vi "Set Framed Sensor Path.vi"(8 "error in (no error)":errorcluster, 10 "Framed Sensor Path":path, 11 "Sensor Model in":refnum<class "Sensor Model.lvclass">) -> (0 "error out":errorcluster, 3 "Sensor Model out":refnum<class "Sensor Model.lvclass">)   [LabVIEW 2013, in "Sensor Model.lvlib" / "Sensor Model.lvclass"]
uses:
  Sensor Model.lvclass
  Sensor Model.lvclass/Sensor Model.ctl
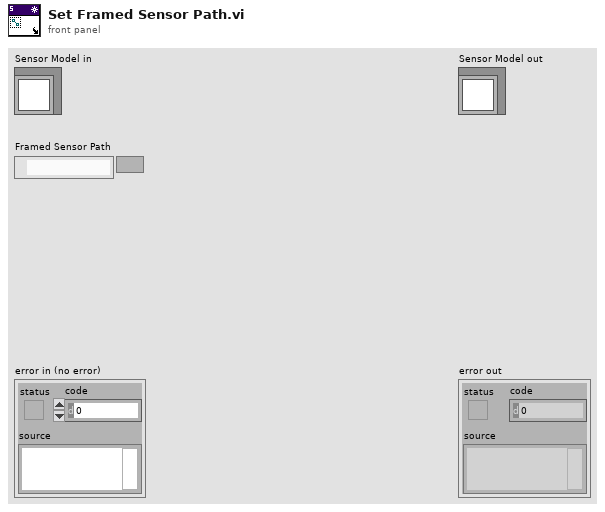
[diagram p1: front panel]
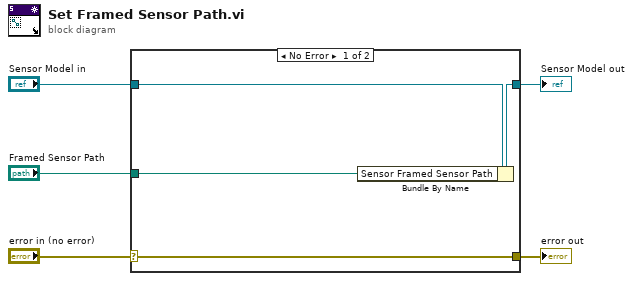
[diagram p0: block diagram]
diagram:
  n1 = case shown="No Error" "error in (no error)" {
    selector: "error in (no error)" -> [w9 w10]
    tunnel: [w9 w10] -> w4
    tunnel: [w7 w11] -> w2
    tunnel: "Sensor Model in" -> [w8 w11]
    tunnel: "Framed Sensor Path" -> [w6 _]
    frame No Error {
      n2 = Bundle By Name(cluster=w8, "Sensor Framed Sensor Path"=w6) -> (w7:refnum<class "Sensor Model.lvclass">)
    }
    frame Error {
    }
  }
  "error out" <- w4
  "Sensor Model out" <- w2
